vi "Build Configuration Frame.vi"(5 "CFG-3 PMU location":T1={"latitude [deg]"=inf, "longitude [deg]"=inf, "elevation [m]"=inf}, 7 "CFG-3 algorithm factors [us]":T2, 8 "error in (no error)":errorcluster, 9 "system info in":refnum<class "PMU System Info.lvclass">, 10 "configuration change count (0)":u16, 11 "configuration frame type":enum16{"CFG-1", "CFG-2", "CFG-3"}(ring)) -> (0 "error out":errorcluster, 1 "system info out":refnum<class "PMU System Info.lvclass">, 3 "configuration frame":string)   [LabVIEW 2014, in "NI_EP_PMU.lvlib"]
doc: "Builds a configuration frame as defined in IEEE Std C37.118.2-2011."
uses:
  <vilib>/addons/Electrical Power/PMU/NI_EP_PMU.lvlib
  <vilib>/addons/Electrical Power/PMU/Common/Classes/PMU System Info/PMU System Info.lvclass
  <vilib>/addons/Electrical Power/PMU/Common/Controls/pmu_CFG-3 Dynamic Response Factors.ctl
  <vilib>/addons/Electrical Power/PMU/Common/Controls/pmu_CFG-3 PMU location.ctl
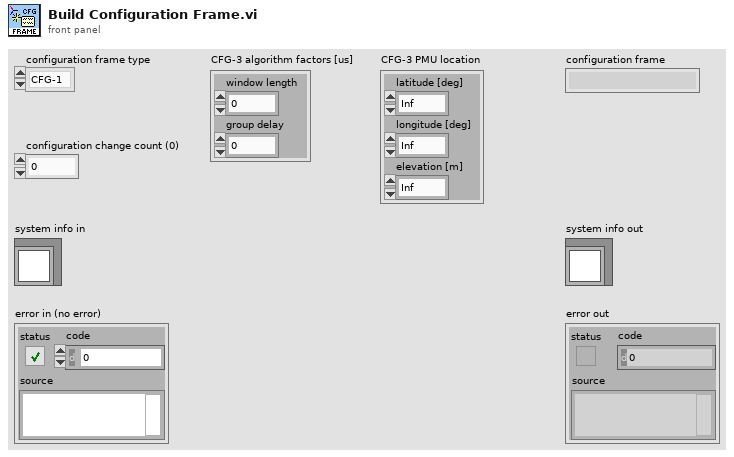
[diagram p1: front panel]
types:
  T1 = typedef "NI_EP_PMU.lvlib/pmu_CFG-3 PMU location.ctl" = cluster{"latitude [deg]":sgl, "longitude [deg]":sgl, "elevation [m]":sgl}
  T2 = typedef "NI_EP_PMU.lvlib/pmu_CFG-3 Dynamic Response Factors.ctl" = cluster{"window length":i32, "group delay":i32}
  T3 = typedef "LVDateTimeRec.ctl" = cluster{"fractional second":dbl, "second":i32, "minute":i32, "hour":i32, "day of month":i32, "month":i32, "year":i32, "day of week":i32, "day of year":i32, "DST":i32}
  T4 = typedef "NI_EP_PMU.lvlib/pmu_CFG Class.ctl" = cluster{"station name":string, "PMU ID":u16, "time base":u32, "nominal frequency":enum16{"50 Hz", "60 Hz"}, "reporting rate":i16, "phasor number":u16, "analog number":u16, "digital number":u16, "channel names":string[], "phasor units":u32[], "analog units":u32[], "digital units":u32[], "data format":u16, "number of PMUs":u16}
  T5 = typedef "NI_EP_PMU.lvlib/pmu_CFG-3 Class.ctl" = cluster{"station name":string, "PMU ID":u16, "global PMU ID":u64, "time base":u32, "nominal frequency":enum16{"50 Hz", "60 Hz"}, "reporting rate":i16, "phasor number":u16, "analog number":u16, "digital number":u16, "channel names":string[], "phasor scale first 4 bytes":u32[], "phasor scale factors":sgl[], "phasor angle offsets [rad]":sgl[], "analog scale factors":sgl[], "analog magnitude offsets":sgl[], "digital units":u32[], "data format":u16, "number of PMUs":u16}
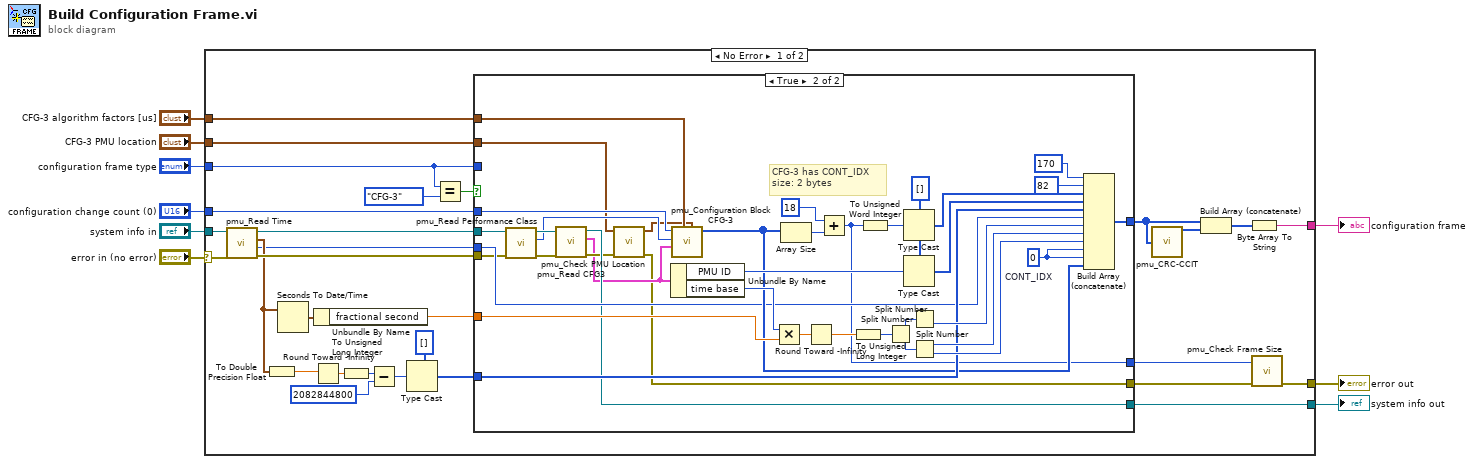
[diagram p0: block diagram]
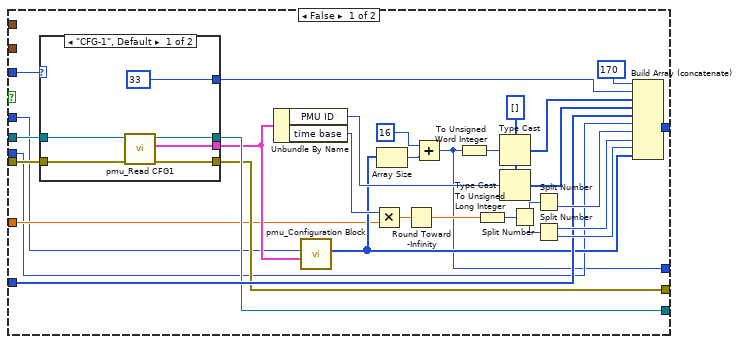
[diagram p2: hidden frame]
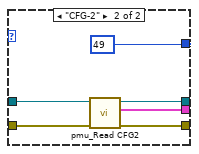
[diagram p3: hidden frame]
diagram:
  n1 = case shown="No Error" "error in (no error)" {
    selector: "error in (no error)" -> [w26 w120]
    tunnel: "system info in" -> [w27 w121]
    tunnel: "configuration change count (0)" -> [w30 _]
    tunnel: "configuration frame type" -> [w18 _]
    tunnel: [w31 _] -> w5
    tunnel: [w16 w121] -> w4
    tunnel: [w13 w120] -> w3
    tunnel: "CFG-3 algorithm factors [us]" -> [w12 _]
    tunnel: "CFG-3 PMU location" -> [w11 _]
    frame No Error {
      n2 = call <vilib>:"pmu_Read Time.vi"("error in (no error)"=w26, "system info in"=w27) -> ("error out"=w24:errorcluster, "time quality"=w20:u8, "time stamp"=w23:timestamp, "system info out"=w25:refnum<class "PMU System Info.lvclass">)  [unwired: 6 in]
      n3 = To Double Precision Float(number=w23) -> (double precision float=w28:dbl)
      n4 = Seconds To Date/Time(time stamp (now)=w23) -> (date time rec=w33:T3)  [unwired: 1 in]
      n5 = Round Toward -Infinity(1:w28) -> (0:w29:dbl)
      n6 = Unbundle By Name(w33) -> ("fractional second"=w21:dbl)
      n7 = To Unsigned Long Integer(number=w29) -> (unsigned 32bit integer=w32:u32)
      n8 = Subtract(x=w32, y=u32 2082844800 ("seconds between 1970.1.1.8:00:00.000 AM and 1904.1.1.12:00:00.000 AM")) -> (x-y=w35:u32)
      n9 = Type Cast(type=u8[] [] ("appended array"), x=w35) -> (*(type *) &x=w34:u8[])
      n10 = Equal?(x=w18, y=enum16{"CFG-1", "CFG-2", "CFG-3"}."CFG-3") -> (x = y?=w19:bool)
      n11 = case shown="True" w19 {
        tunnel: [w62 w105] -> w37
        tunnel: w34 -> [w59 w104]
        tunnel: w18 -> [w54 _]
        tunnel: [w53 w90] -> w16
        tunnel: [w52 w85] -> w14
        tunnel: w30 -> [w42 w99]
        tunnel: w25 -> [w46 w94]
        tunnel: w24 -> [w45 w95]
        tunnel: w21 -> [w44 w111]
        tunnel: w20 -> [w43 w96]
        tunnel: w12 -> [_ w97]
        tunnel: w11 -> [_ w89]
        tunnel: [w39 w82] -> w10
        frame False {
          w58 = u8[] [] ("appended array")
          n12 = case shown="\"CFG-1\", Default" w54 {
            tunnel: [w75 w76] -> w53
            tunnel: [w74 w78] -> w52
            tunnel: [w73 w77] -> w51
            tunnel: [u8 33 ("element") u8 49 ("element")] -> w49
            tunnel: w45 -> [w71 w79]
            tunnel: w46 -> [w70 w80]
            frame "CFG-1", Default {
              n13 = call <vilib>:"pmu_Read CFG1.vi"("error in (no error)"=w71, "system info in"=w70) -> ("error out"=w74:errorcluster, "CFG-1"=w73:T4, "system info out"=w75:refnum<class "PMU System Info.lvclass">)  [unwired: 7 in]
            }
            frame "CFG-2" {
              n14 = call <vilib>:"pmu_Read CFG2.vi"("error in (no error)"=w79, "system info in"=w80) -> ("error out"=w78:errorcluster, "CFG-2"=w77:T4, "system info out"=w76:refnum<class "PMU System Info.lvclass">)  [unwired: 7 in]
            }
          }
          n15 = Unbundle By Name(w51) -> ("PMU ID"=w56:u16, "time base"=w55:u32)
          n16 = call <vilib>:"pmu_Configuration Block.vi"("CFG class"=w51, "configuration change count"=w42) -> ("data"=w50:u8[])  [unwired: 9 in]
          n17 = Multiply(x=w55, y=w44) -> (x*y=w48:dbl)
          n18 = Array Size(array=w50) -> (size(s)=w41:i32)
          n19 = Round Toward -Infinity(1:w48) -> (0:w47:dbl)
          n20 = Add(x=16 ("y"), y=w41) -> (x+y=w39:i32)
          n21 = To Unsigned Word Integer(number=w39) -> (unsigned 16bit integer=w40:u16)
          n22 = To Unsigned Long Integer(number=w47) -> (unsigned 32bit integer=w57:u32)
          n23 = Type Cast(type=w58, x=w40) -> (*(type *) &x=w61:u8[])
          n24 = Type Cast(type=w58, x=w56) -> (*(type *) &x=w60:u8[])
          n25 = Split Number(x=w57) -> (hi(x)=w66:u16, lo(x)=w67:u16)
          n26 = Split Number(x=w66) -> (lo(x)=w65:u8)  [unwired: 1 out]
          n27 = Split Number(x=w67) -> (hi(x)=w64:u8, lo(x)=w63:u8)
          n28 = Build Array (concatenate)(u8 170 ("element"), w49, w61, w60, w59, w43, w65, w64, w63, w50) -> (w62:u8[])
        }
        frame True {
          w98 = u8 0  # CONT_IDX
          w106 = u8[] [] ("appended array")
          # "CFG-3 has CONT_IDX\nsize: 2 bytes"
          n29 = call <vilib>:"pmu_Read Performance Class.vi"("error in (no error)"=w95, "system info in"=w94) -> ("error out"=w91:errorcluster, "performance class"=w92:enum8{"M Class", "P Class"}, "system info out"=w93:refnum<class "PMU System Info.lvclass">)  [unwired: 7 in]
          n30 = call <vilib>:"pmu_Read CFG3.vi"("error in (no error)"=w91, "system info in"=w93) -> ("error out"=w88:errorcluster, "CFG-3"=w86:T5, "system info out"=w90:refnum<class "PMU System Info.lvclass">)  [unwired: 7 in]
          n31 = call <vilib>:"pmu_Check PMU Location.vi"("error in (no error)"=w88, "CFG-3 PMU location"=w89) -> ("error out"=w85:errorcluster, "CFG-3 PMU location"=w87:T1)  [unwired: 8 in]
          n32 = Unbundle By Name(w86) -> ("PMU ID"=w101:u16, "time base"=w110:u32)
          n33 = call <vilib>:"pmu_Configuration Block CFG-3.vi"("CFG-3 PMU location"=w87, "CFG-3 dynamci response factors [us]"=w97, "CFG-3 class"=w86, "performance class"=w92, "configuration change count"=w99) -> ("data"=w100:u8[])  [unwired: 6 in]
          n34 = Multiply(x=w110, y=w111) -> (x*y=w113:dbl)
          n35 = Array Size(array=w100) -> (size(s)=w84:i32)
          n36 = Round Toward -Infinity(1:w113) -> (0:w112:dbl)
          n37 = Add(x=18 ("y"), y=w84) -> (x+y=w82:i32)
          n38 = To Unsigned Long Integer(number=w112) -> (unsigned 32bit integer=w114:u32)
          n39 = To Unsigned Word Integer(number=w82) -> (unsigned 16bit integer=w83:u16)
          n40 = Split Number(x=w114) -> (hi(x)=w115:u16, lo(x)=w116:u16)
          n41 = Type Cast(type=w106, x=w83) -> (*(type *) &x=w102:u8[])
          n42 = Type Cast(type=w106, x=w101) -> (*(type *) &x=w103:u8[])
          n43 = Split Number(x=w115) -> (lo(x)=w109:u8)  [unwired: 1 out]
          n44 = Split Number(x=w116) -> (hi(x)=w108:u8, lo(x)=w107:u8)
          n45 = Build Array (concatenate)(u8 170 ("element"), u8 82 ("element"), w102, w103, w104, w96, w109, w108, w107, w98, w98, w100) -> (w105:u8[])
        }
      }
      n46 = call <vilib>:"pmu_CRC-CCIT.vi"("byte array"=w37) -> ("CRCbytes"=w36:u8[])  [unwired: 13 in, 1 out]
      n47 = Build Array (concatenate)(w37, w36) -> (w15:u8[])
      n48 = Byte Array To String(unsigned byte array=w15) -> (string=w31:string)
      n49 = call <vilib>:"pmu_Check Frame Size.vi"("error in (no error)"=w14, "frame size"=w10) -> ("error out"=w13:errorcluster)  [unwired: 9 in]
    }
    frame Error {
    }
  }
  "configuration frame" <- w5
  "error out" <- w3
  "system info out" <- w4
